vi "Send Message - Stop.vi"(8 "error in (no error)":errorcluster) -> (0 "error out":errorcluster)   [LabVIEW 2010, in "Template Module.lvlib"]
doc: "Sends a Stop message to the Module loop"
uses:
  Template Module.lvlib
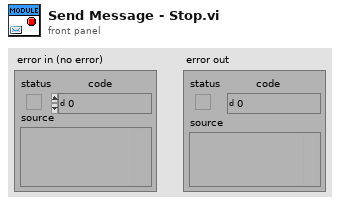
[diagram p1: front panel]
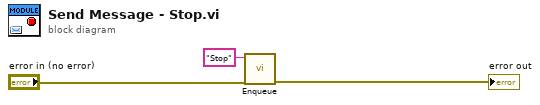
[diagram p0: block diagram]
diagram:
  n1 = call "Enqueue.vi"("error in (no error)"="error in (no error)", "Message"="Stop") -> ("error out"=→"error out":errorcluster)  [unwired: 9 in]
